vi "Get ObjectType.vi"(8 "error in":errorcluster, 11 "VAR in":refnum<class "VAR.lvclass">) -> (0 "error out":errorcluster, 1 "Defined?":bool, 2 "ObjectType":T1 items=["UNKNOWN"=255, "NULL"=0, "DOMAIN"=2, "DEFTYPE"=5, "DEFSTRUCT"=6, "VAR"=7, "ARRAY"=8, "RECORD"=9], 3 "VAR out":refnum<class "VAR.lvclass">)   [LabVIEW 2019, in "Electronic Datasheet.lvlib" / "VAR.lvclass"]
uses:
  VAR.lvclass
  Object Type/Object Type Base.lvclass
  Object Type.ctl
  Electronic Datasheet.lvlib
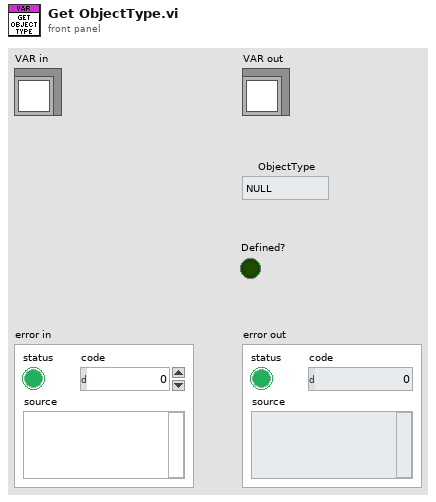
[diagram p1: front panel]
types:
  T1 = typedef "Electronic Datasheet.lvlib/Object Type.ctl" = u8
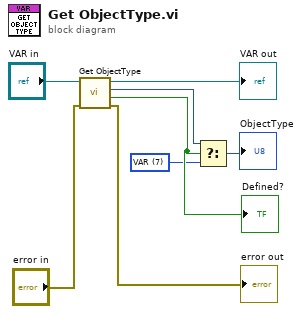
[diagram p0: block diagram]
diagram:
  w1 = T1 7 items=["NULL"=0, "DOMAIN"=2, "DEFTYPE"=5, "DEFSTRUCT"=6, "VAR"=7, "ARRAY"=8, "RECORD"=9] ("ObjectType")
  n1 = call-parent "Get ObjectType.vi"("error in"="error in", "Object Type in"="VAR in") -> ("error out"=→"error out":errorcluster, "Defined?"=w2:bool, "ObjectType"=w4:T1, "Object Type out"=→"VAR out":refnum<class "VAR.lvclass">)  [unwired: 6 in]
  "Defined?" <- w2
  n2 = Select(t=w4, s=w2, f=w1) -> (s? t:f=→"ObjectType":T1)
